vi "DWF MSO Enable Digital Channels.vi"(0 "Instrument Handle In":u32, 1 "Enable Channel":bool, 5 "Channel":string, 11 "Error In":errorcluster caption="Error In (no error)") -> (4 "Instrument Handle Out":u32, 15 "Error Out":errorcluster)   [LabVIEW 2015, in "DigilentWF.lvlib"]
doc: "Enables or disables the specified digital channels."
uses:
  <vilib>/DigilentWF/DigilentWF.lvlib
  dwf.dll
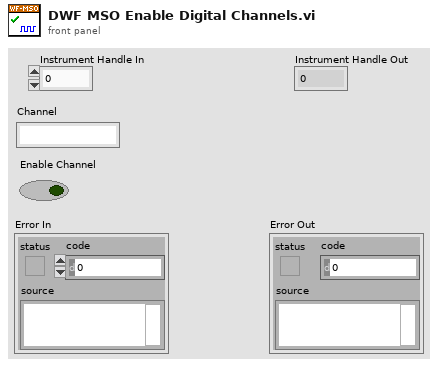
[diagram p1: front panel]
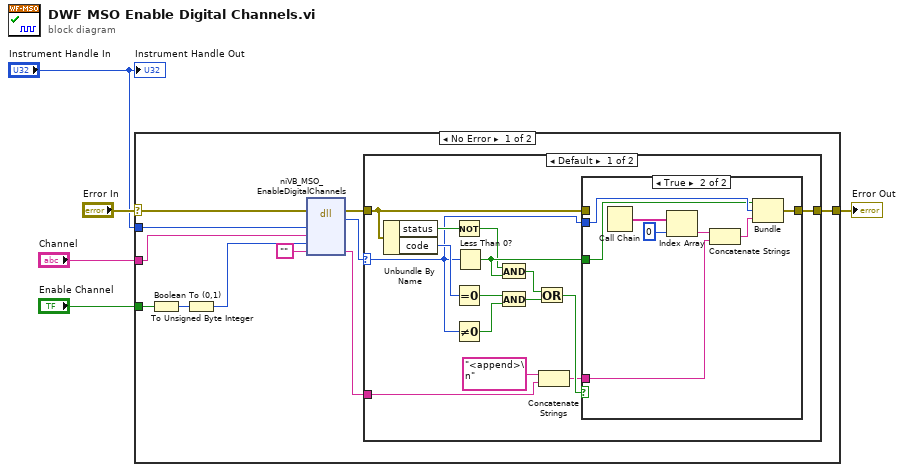
[diagram p0: block diagram]
diagram:
  n1 = case "outter_case" shown="No Error" "Error In" {
    selector: "Error In" -> [w16 w42]
    tunnel: [w13 w42] -> w4
    tunnel: "Instrument Handle In" -> [w12 _]
    tunnel: "Enable Channel" -> [w10 _]
    tunnel: "Channel" -> [w6 _]
    frame No Error {
      n2 = Boolean To (0,1)(Boolean=w10) -> (0, 1=w11:i16)
      n3 = To Unsigned Byte Integer(number=w11) -> (unsigned 8bit integer=w9:u8)
      n4 = dll-call lib="dwf.*" fn="niVB_MSO_EnableDigitalChannels"(error in=w16, "InstrumentHandle"=w12, "Channel"=w6, "EnableChannel"=w9, "szError"="") -> (error out=w15:errorcluster, "return type"=w14:i32, "szError"=w7:string)  [unwired: 5 in, 1 out]
      n5 = case "inner_case" shown="Default" w14 {
        selector: w14 -> [w21 _]
        tunnel: w15 -> [w22 w41]
        tunnel: [w18 w41] -> w13
        tunnel: w7 -> [w17 _]
        frame Default {
          n6 = Unbundle By Name(w22) -> ("status"=w26:bool, "code"=w30:i32)
          n7 = Not(x=w26) -> (.not. x?=w29:bool)
          n8 = Equal To 0?(x=w30) -> (x = 0?=w25:bool)
          n9 = Not Equal To 0?(x=w21) -> (x != 0?=w28:bool)
          n10 = Less Than 0?(x=w21) -> (x < 0?=w31:bool)
          n11 = And(x=w29, y=w31) -> (x .and. y?=w27:bool)
          n12 = And(x=w25, y=w28) -> (x .and. y?=w24:bool)
          n13 = Or(x=w27, y=w24) -> (x .or. y?=w23:bool)
          n14 = Concatenate Strings("<append>\n" ("string"), w17) -> (w20:string)
          n15 = case shown="True" w23 {
            tunnel: [w32 w39] -> w18
            tunnel: w21 -> [_ w38]
            tunnel: w31 -> [_ w37]
            tunnel: w22 -> [w32 _]
            tunnel: w20 -> [_ w33]
            frame False {
            }
            frame True {
              n16 = Call Chain() -> (call chain=w36:string[])
              n17 = Index Array(array=w36, index=0) -> (element=w35:string)
              n18 = Concatenate Strings(w35, w33) -> (w40:string)
              n19 = Bundle(w37, "return type"=w38, w40) -> (w39:cluster{bool, "return type":i32, string})  [unwired: 1 out]
            }
          }
        }
        frame 0 {
        }
      }
    }
    frame Error {
    }
  }
  "Error Out" <- w4
  "Instrument Handle Out" <- "Instrument Handle In"
